vi "HapticIO_9.vi"() -> ()   [LabVIEW 2017]
uses:
  Control 3.ctl
  Control 4.ctl
  Control 5.ctl
  Control 1.ctl
  Control 2.ctl
  <vilib>/Utility/file.llb/Read Delimited Spreadsheet (DBL).vi
  <userlib>/PositionDLL/PositionDLL.lvlib
panel:
  out "New Output":dbl
  out "pnz":dbl
  out "pny":dbl
  out "pnx":dbl
  out "pd":dbl
  out "CLICK":dbl
  in  "START":bool
  in  "STOP":bool
  in  "Resolution:":T1=1590.0
  out "Output":dbl
  in  "Sensitivity":T2=3.5
  in  "size:":T3=300.0
  in  "zi:":T4=380.0
  in  "xi:":T5=950.0
  out "psi":dbl
  out "phi":dbl
  out "theta":dbl
  out "Fz":dbl
  out "Fy":dbl
  out "Fx":dbl
  out "z":dbl
  out "y":dbl
  out "x":dbl
  # "Sample Window"
  # "Position"
  # "Force"
  # "Angles"
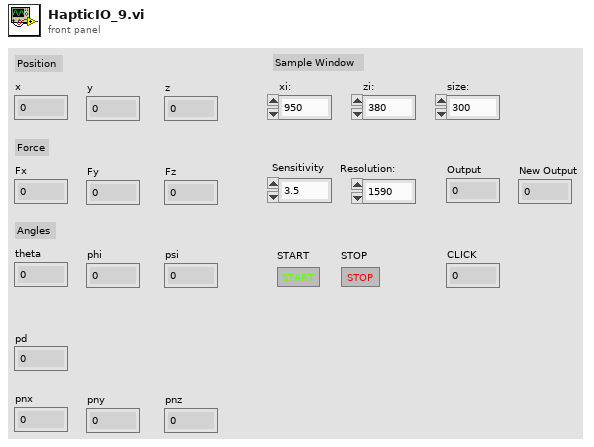
[diagram p1: front panel]
types:
  T1 = typedef "Control 2.ctl" = dbl
  T2 = typedef "Control 1.ctl" = dbl
  T3 = typedef "Control 5.ctl" = dbl
  T4 = typedef "Control 4.ctl" = dbl
  T5 = typedef "Control 3.ctl" = dbl
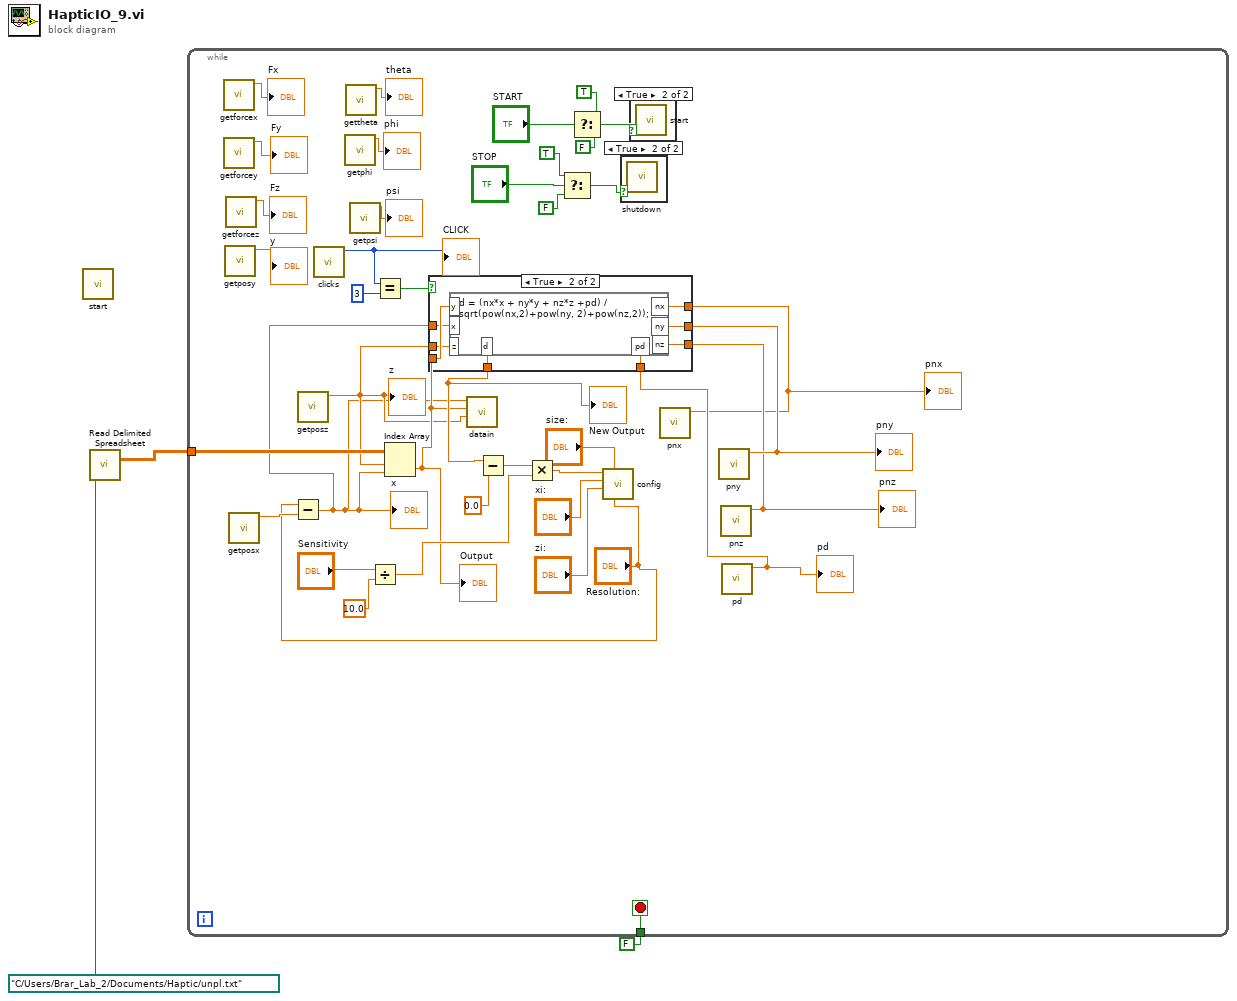
[diagram p0: block diagram]
diagram:
  n1 = call <userlib>:"start.vi"() -> ()  [unwired: 11 in, 1 out]
  n2 = call-poly <vilib>:"Read Delimited Spreadsheet.vi"("file path (dialog if empty)"=path "C:/Users/Brar_Lab_2/Documents/Haptic/unpl.txt") -> ("all rows"=w2:dbl[][])  [unwired: 9 in, 5 out]
  n3 = while {
    tunnel: FALSE -> [w42]
    tunnel: w2 -> [w41]
    stop <- w42 stop-if-true
    n4 = call <userlib>:"getforcex.vi"() -> ("function return"=→"Fx":dbl)  [unwired: 11 in]
    n5 = call <userlib>:"getforcey.vi"() -> ("function return"=→"Fy":dbl)  [unwired: 11 in]
    n6 = call <userlib>:"getposy.vi"() -> ("function return"=→"y":dbl)  [unwired: 11 in]
    n7 = call <userlib>:"getforcez.vi"() -> ("function return"=→"Fz":dbl)  [unwired: 11 in]
    n8 = call <userlib>:"getposx.vi"() -> ("function return"=w9:dbl)  [unwired: 11 in]
    n9 = Subtract(x="Resolution:", y=w9) -> (x-y=w5:T1)
    "x" <- w5
    n10 = call <userlib>:"getposz.vi"() -> ("function return"=w7:dbl)  [unwired: 11 in]
    "z" <- w7
    n11 = call <userlib>:"clicks.vi"() -> ("function return"=w13:i32)  [unwired: 11 in]
    "CLICK" <- w13
    n12 = call <userlib>:"getphi.vi"() -> ("function return"=→"phi":dbl)  [unwired: 11 in]
    n13 = call <userlib>:"gettheta.vi"() -> ("function return"=→"theta":dbl)  [unwired: 11 in]
    n14 = call <userlib>:"getpsi.vi"() -> ("function return"=→"psi":dbl)  [unwired: 11 in]
    n15 = Divide(x="Sensitivity", y=10.0) -> (x/y=w28:T2)
    n16 = Equal?(x=w13, y=3) -> (x = y?=w11:bool)
    n17 = Index Array(array=w41, index (row)=w7, index (col)=w5) -> (element=w8:dbl)
    "Output" <- w8
    n18 = call <userlib>:"datain.vi"("zin"=w7, "output"=w8, "xin"=w5) -> ()  [unwired: 9 in]
    n19 = Select(t=TRUE, s="STOP", f=FALSE) -> (s? t:f=w21:bool)
    n20 = Select(t=TRUE, s="START", f=FALSE) -> (s? t:f=w17:bool)
    n21 = case shown="True" w21 {
      frame False {
      }
      frame True {
        n22 = call <userlib>:"shutdown.vi"() -> ()  [unwired: 12 in]
      }
    }
    n23 = case shown="True" w17 {
      frame False {
      }
      frame True {
        n24 = call <userlib>:"start.vi"() -> ()  [unwired: 11 in, 1 out]
      }
    }
    n25 = call <userlib>:"pnx.vi"() -> ("function return"=w4:dbl)  [unwired: 11 in]
    "pnx" <- w4
    n26 = call <userlib>:"pny.vi"() -> ("function return"=w16:dbl)  [unwired: 11 in]
    "pny" <- w16
    n27 = call <userlib>:"pnz.vi"() -> ("function return"=w15:dbl)  [unwired: 11 in]
    "pnz" <- w15
    n28 = call <userlib>:"pd.vi"() -> ("function return"=w14:dbl)  [unwired: 11 in]
    "pd" <- w14
    n29 = case shown="True" w11 {
      tunnel: w8 -> [w43 w51]
      tunnel: w5 -> [_ w50]
      tunnel: w7 -> [_ w49]
      tunnel: [w43 w48] -> w10
      tunnel: w4 -> [_ w47]
      tunnel: w16 -> [_ w46]
      tunnel: w15 -> [_ w45]
      tunnel: w14 -> [_ w44]
      frame False {
      }
      frame True {
        n30 = formula code="d = (nx*x + ny*y + nz*z +pd) / sqrt(pow(nx,2)+pow(ny, 2)+pow(nz,2));"("y"=w51, "z"=w49, "x"=w50, "nx"=w47, "ny"=w46, "nz"=w45, "pd"=w44) -> ("d"=w48:dbl)
      }
    }
    "New Output" <- w10
    n31 = Subtract(x=w10, y=0.0 ("x")) -> (x-y=w39:dbl)
    n32 = Multiply(x=w39, y=w28) -> (x*y=w38:T2)
    n33 = call <userlib>:"config.vi"("imagesize"="Resolution:", "scope"="size:", "z0"="zi:", "x0"="xi:", "ypos"=w38) -> ()  [unwired: 7 in]
  }
